vi "Get Pre Amp Gain.vi"(10 "gain":sgl, 11 "index":i32) -> (2 "gain out":sgl, 3 "function return":u32)   [LabVIEW 2018, in "Copy of Andor SDK.lvlib"]
doc: "EXPNETTYPE unsigned int WINAPI GetPreAmpGain(int index, float * gain);"
uses:
  Copy of Andor SDK.lvlib
  <userlib>/Andor SDK/ATMCD32D.dll
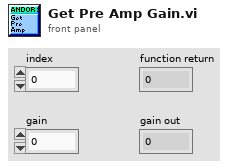
[diagram p1: front panel]
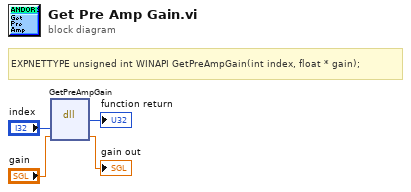
[diagram p0: block diagram]
diagram:
  # "EXPNETTYPE unsigned int WINAPI GetPreAmpGain(int index, float * gain);"
  n1 = dll-call lib="C:/Program Files (x86)/National Instruments/LabVIEW 2018/user.lib/Andor SDK/ATMCD32D.*" fn="GetPreAmpGain"("index"="index", "gain"="gain") -> (→"function return":u32, "gain"=→"gain out":sgl)  [unwired: 4 in, 2 out]
